vi "Build DIO Section.vi"(6 "Cancelled?":bool, 8 "error in (no error)":errorcluster, 9 "Card Position in":T1 {"Slot #" max=15}, 10 "Name in":string, 11 "Node Ptr in":u64) -> (0 "error out":errorcluster)   [LabVIEW 2014, in "SLSC configuration System Explorer.lvlib"]
uses:
  SLSC configuration System Explorer.lvlib
  Type Defs/Card Position.ctl
  Shared/SPI Utility/Slot #.ctl
  Shared/Constants.vi
  <vilib>/NI Veristand/Custom Device API/Custom Device API.lvlib
  Shared/SLSC configuration Shared.lvlib
  <vilib>/NI Veristand/Custom Device Tools/Custom Device Utility Library/Custom Device Utility Library.lvlib
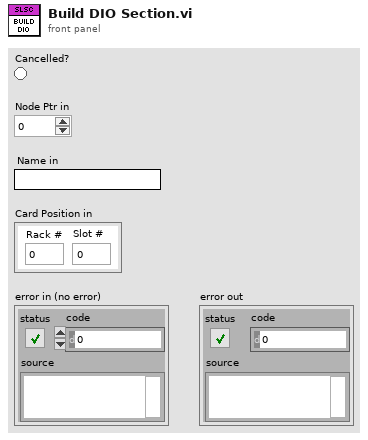
[diagram p1: front panel]
types:
  T1 = typedef "SLSC configuration Shared.lvlib/Card Position.ctl" = cluster{"Rack #":u8, "Slot #":T2}
  T2 = typedef "SLSC configuration Shared.lvlib/Slot #.ctl" = u8
  T3 = typedef "Custom Device API.lvlib/Custom Device Item Ref.ctl" = u64
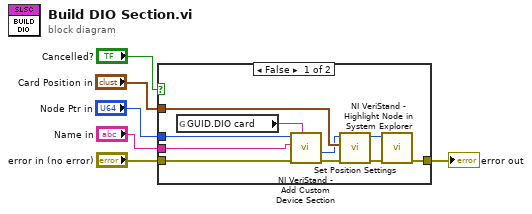
[diagram p0: block diagram]
diagram:
  n1 = case shown="False" "Cancelled?" {
    tunnel: "error in (no error)" -> [w15 w17]
    tunnel: "Name in" -> [w14 _]
    tunnel: "Node Ptr in" -> [w13 _]
    tunnel: "Card Position in" -> [w11 _]
    tunnel: [w12 w17] -> w5
    frame False {
      n2 = global read "Constants.vi" "GUID.DIO card"() -> (w16:string)
      n3 = call <vilib>:"NI VeriStand - Add Custom Device Section.vi"("GUID (Default Section)"=w16, "error in (no error)"=w15, "Section Name"=w14, "Parent Ref in"=w13) -> ("error out"=w10:errorcluster, "Section Ptr"=w7:T3)  [unwired: 4 in, 2 out]
      n4 = call "Set Position Settings.vi"("error in (no error)"=w10, "Card Position"=w11, "Item Ref in"=w7) -> ("error out"=w9:errorcluster, "Item Ref out"=w8:T3)  [unwired: 7 in]
      n5 = call <vilib>:"NI VeriStand - Highlight Node in System Explorer.vi"("error in (no error)"=w9, "Item Ref in"=w8) -> ("error out"=w12:errorcluster)  [unwired: 8 in, 1 out]
    }
    frame True {
    }
  }
  "error out" <- w5
